vi "系统设置_古田污水厂.vi"() -> ()   [LabVIEW 2016]
uses:
  <vilib>/Utility/miscctls.llb/LVPointTypeDef.ctl
  <vilib>/Utility/config.llb/Read Key (U32).vi
  <vilib>/Utility/config.llb/Write Key (I32).vi
  PLC/PLC.lvlib
  <vilib>/ptbypt/NI_PtbyPt.lvlib
  <vilib>/Utility/config.llb/NI_LVConfig.lvlib
panel:
  out "循环次数":i32
  out "CODCr启动失败":bool
  out "输出簇":T1
  in  "运行模式":enum16{"维护模式", "常规模式", "应急模式", "质控模式"}(ring)
  in  "运行周期":i16=4 caption="运行间隔" min=1 max=24
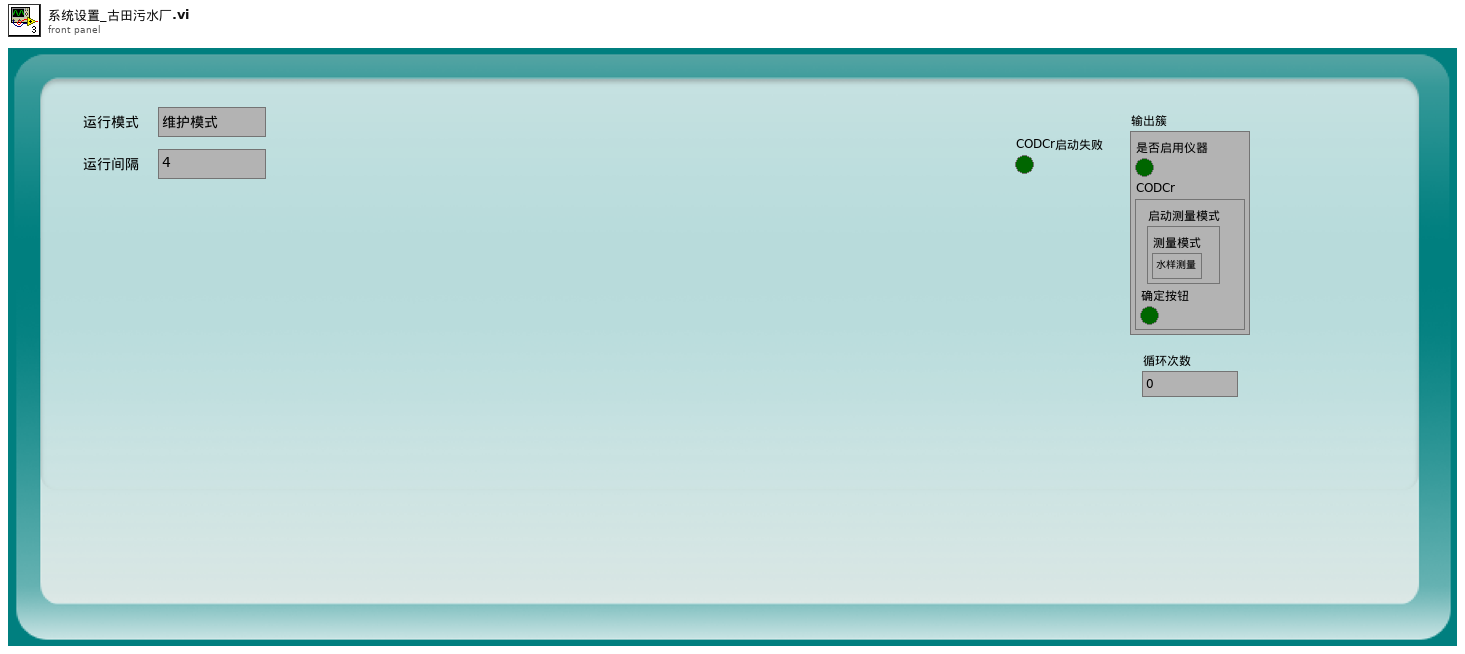
[diagram p1: front panel]
types:
  T1 = cluster{"是否启用仪器":bool, "CODCr":cluster{"启动测量模式":cluster{"测量模式":enum16{"水样测量", "标样核查", "零点核查", "加标回收", "平行样", "校零", "校标"}}, "确定按钮":bool}}
  T2 = typedef "LVPointTypeDef.ctl" = cluster{"Horizontal":i16, "Vertical":i16}
  T3 = typedef "NI_LVConfig.lvlib/Config Data RefNum.ctl" = refnum<k1>
  T4 = enum16{"水样测量", "标样核查", "零点核查", "加标回收", "平行样", "校零", "校标"}
  T5 = typedef "LVDateTimeRec.ctl" = cluster{"秒数的小数部分":dbl, "秒":i32, "分":i32, "时":i32, "日":i32, "月":i32, "年":i32, "天数（周）":i32, "天数（年）":i32, "DST":i32}
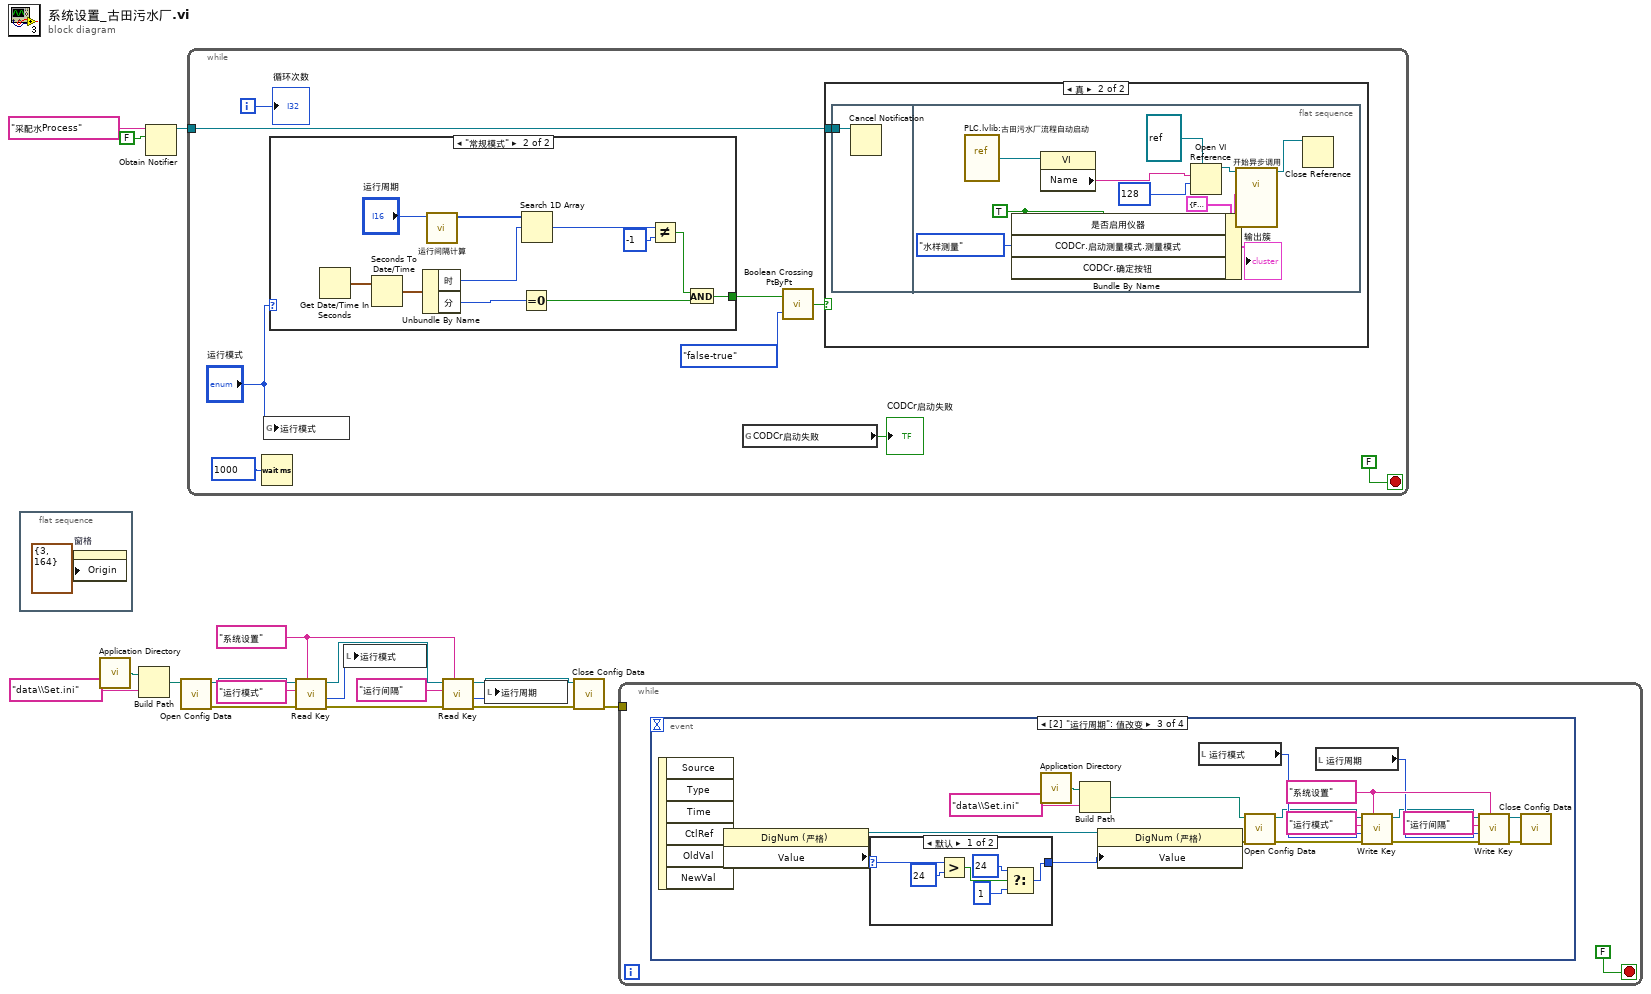
[diagram p0: block diagram]
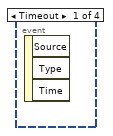
[diagram p4: hidden frame]
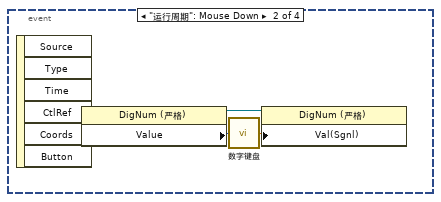
[diagram p5: hidden frame]
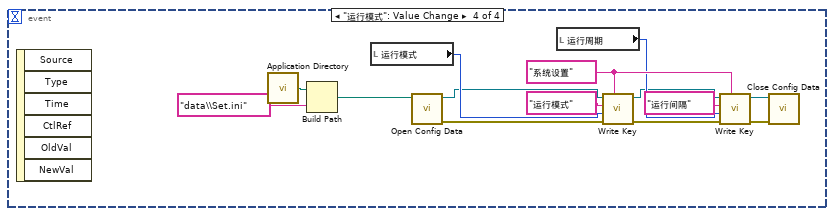
[diagram p7: hidden frame]
diagram:
  w2 = "系统设置" ("section")
  n1 = flat-sequence {
    frame #0 {
      n2 = property on="窗格" class="Pane"("Origin"=T2 {"Horizontal"=3, "Vertical"=164} ("原点")) -> ()  [unwired: 2 in, 2 out]
    }
  }
  n3 = call <vilib>:"Application Directory.vi"() -> ("Application Directory"=w13:path)
  n4 = Build Path(base path=w13, name or relative path="data\\Set.ini" ("名称或相对路径")) -> (appended path=w11:path)
  n5 = Obtain Notifier(name (unnamed)="采配水Process" ("名称（未命名）"), notification data type=FALSE) -> (notifier out=w16:refnum<notifier>)  [unwired: 2 in, 2 out]
  n6 = call <vilib>:"Open Config Data.vi"("configuration file path"=w11) -> ("error out"=w14:errorcluster, "refnum"=w15:T3)  [unwired: 8 in, 1 out]
  n7 = while {
    tunnel: w16 -> [w26]
    i -> [w20]
    stop <- FALSE stop-if-true
    n8 = Wait (ms)(milliseconds to wait=u32 1000 ("等待时间（毫秒）")) -> ()  [unwired: 1 out]
    n9 = global write "系统变量.vi" "运行模式"("运行模式") -> ()
    n10 = case shown="\"常规模式\"" "运行模式" {
      tunnel: [_ w41] -> w25
      frame "维护模式", Default {
      }
      frame "常规模式" {
        n11 = Get Date/Time In Seconds() -> (seconds since 1Jan1904=w50:timestamp)
        n12 = Seconds To Date/Time(time stamp (now)=w50) -> (date time rec=w49:T5)  [unwired: 1 in]
        n13 = Unbundle By Name(w49) -> ("时"=w46:i32, "分"=w48:i32)
        n14 = call "运行间隔计算.vi"("运行周期"="运行周期") -> ("数组"=w47:i32[])  [unwired: 10 in]
        n15 = Equal To 0?(x=w48) -> (x = 0?=w42:bool)
        n16 = Search 1D Array(1D array=w47, element=w46) -> (index of element=w45:i32)  [unwired: 1 in]
        n17 = Not Equal?(x=w45, y=-1) -> (x != y?=w43:bool)
        n18 = And(x=w43, y=w42) -> (x .and. y?=w41:bool)
      }
    }
    n19 = global read "系统变量.vi" "CODCr启动失败"() -> (→"CODCr启动失败":bool)
    n20 = call <vilib>:"Boolean Crossing PtByPt.vi"("direction"=enum16{"either", "false-true", "true-false"}."false-true", "input"=w25) -> ("crossing"=w23:bool)  [unwired: 1 in]
    n21 = case shown="真" w23 {
      tunnel: w26 -> [_ w29]
      frame False {
      }
      frame True {
        n22 = flat-sequence {
          tunnel: w29 -> [w30]
          frame #0 {
            n23 = Cancel Notification(0:w30) -> ()  [unwired: 1 in, 3 out]
          }
          frame #1 {
            w38 = TRUE ("是否启用仪器")
            n24 = vi-ref "PLC.lvlib:古田污水厂流程自动启动.vi"() -> (w32:refnum<vi>)
            n25 = Bundle By Name(cluster=T1 {"是否启用仪器"=FALSE, "CODCr"={"启动测量模式"={"测量模式"=enum."水样测量"}, "确定按钮"=TRUE}} ("参数"), "是否启用仪器"=w38, "CODCr.启动测量模式.测量模式"=T4."水样测量", "CODCr.确定按钮"=w38) -> (w33:T1)
            "输出簇" <- w33
            n26 = property class="VI"(reference=w32) -> ("Name"=w31:string)  [unwired: 1 in, 2 out]
            n27 = Open VI Reference(type specifier VI Refnum (for type only)=refnum<vi> refnum ("类型说明符VI引用句柄（仅用于类型）"), vi path=w31, options=128 ("选项")) -> (vi reference=w36:refnum<vi>)  [unwired: 3 in, 1 out]
            n28 = call-by-ref "开始异步调用"(reference=w36, "参数"=w33) -> (reference out=w35:refnum<vi>)  [unwired: 11 in, 2 out]
            n29 = Close Reference(reference=w35) -> ()  [unwired: 1 in, 1 out]
          }
        }
      }
    }
    "循环次数" <- w20
  }
  n30 = call-poly <vilib>:"Read Key.vi"("section"=w2, "error in (no error)"=w14, "key"="运行模式" ("section"), "refnum"=w15) -> ("error out"=w7:errorcluster, "value"=w10:u32, "refnum out"=w9:T3)  [unwired: 4 in, 1 out]
  n31 = local write "运行模式"(w10) -> ()
  n32 = call-poly <vilib>:"Read Key.vi"("section"=w2, "error in (no error)"=w7, "key"="运行间隔" ("section"), "refnum"=w9) -> ("error out"=w6:errorcluster, "value"=w3:u32, "refnum out"=w8:T3)  [unwired: 4 in, 1 out]
  n33 = local write "运行周期"(w3) -> ()
  n34 = call <vilib>:"Close Config Data.vi"("error in (no error)"=w6, "refnum"=w8) -> ("error out"=w1:errorcluster)  [unwired: 8 in, 1 out]
  n35 = while {
    tunnel: w1 -> [_]
    stop <- FALSE stop-if-true
    n36 = event shown="[2] \"运行周期\": 值改变" {
      selector: _ -> [_ _ _ _]
      dyn-events: _ -> [_ _ _ _]
      timeout: _ -> [_ _ _ _]
      event Timeout {
        n37 = event-data() -> ()  [unwired: 1 in, 3 out]
      }
      event "运行周期": Mouse Down {
        n38 = event-data() -> ("CtlRef"=w53:refnum<vi>)  [unwired: 1 in, 5 out]
        n39 = property class="DigNum (严格)"(reference=w53) -> (reference out=w55:refnum<vi>, "Value"=w54:i16)  [unwired: 1 in, 1 out]
        n40 = call "数字键盘.vi"("OldNumber"=w54) -> ("NewNumber"=w56:sgl)
        n41 = property class="DigNum (严格)"(reference=w55, "Val(Sgnl)"=w56) -> ()  [unwired: 1 in, 2 out]
      }
      event "运行周期": Value Change {
        w71 = "系统设置" ("section")
        n42 = event-data() -> ("CtlRef"=w75:refnum<vi>)  [unwired: 1 in, 5 out]
        n43 = property class="DigNum (严格)"(reference=w75) -> (reference out=w73:refnum<vi>, "Value"=w74:i16)  [unwired: 1 in, 1 out]
        n44 = case shown="默认" w74 {
          selector: w74 -> [w78 w82]
          tunnel: [w77 w82] -> w72
          frame Default {
            n45 = Greater?(x=w78, y=i16 24) -> (0:w80:bool)
            n46 = Select(t=i16 24 ("y"), s=w80, f=i16 1) -> (s? t:f=w77:i16)
          }
          frame 1..24 {
          }
        }
        n47 = call <vilib>:"Application Directory.vi"() -> ("Application Directory"=w66:path)
        n48 = Build Path(base path=w66, name or relative path="data\\Set.ini" ("名称或相对路径")) -> (appended path=w64:path)
        n49 = property class="DigNum (严格)"(reference=w73, "Value"=w72) -> (error out=w57:errorcluster)  [unwired: 1 in, 1 out]
        n50 = local read "运行模式"() -> (w69:enum16{"维护模式", "常规模式", "应急模式", "质控模式"})
        n51 = call <vilib>:"Open Config Data.vi"("error in (no error)"=w57, "configuration file path"=w64) -> ("error out"=w67:errorcluster, "refnum"=w68:T3)  [unwired: 7 in, 1 out]
        n52 = local read "运行周期"() -> (w70:i16)
        n53 = call-poly <vilib>:"Write Key.vi"("section"=w71, "error in (no error)"=w67, "value"=w69, "key"="运行模式" ("section"), "refnum"=w68) -> ("error out"=w61:errorcluster, "refnum out"=w63:T3)  [unwired: 4 in, 1 out]
        n54 = call-poly <vilib>:"Write Key.vi"("section"=w71, "error in (no error)"=w61, "value"=w70, "key"="运行间隔" ("section"), "refnum"=w63) -> ("error out"=w60:errorcluster, "refnum out"=w62:T3)  [unwired: 4 in, 1 out]
        n55 = call <vilib>:"Close Config Data.vi"("error in (no error)"=w60, "refnum"=w62) -> ()  [unwired: 8 in, 2 out]
      }
      event "运行模式": Value Change {
        w96 = "系统设置" ("section")
        n56 = event-data() -> ()  [unwired: 1 in, 6 out]
        n57 = call <vilib>:"Application Directory.vi"() -> ("Application Directory"=w91:path)
        n58 = Build Path(base path=w91, name or relative path="data\\Set.ini" ("名称或相对路径")) -> (appended path=w89:path)
        n59 = local read "运行模式"() -> (w94:enum16{"维护模式", "常规模式", "应急模式", "质控模式"})
        n60 = call <vilib>:"Open Config Data.vi"("configuration file path"=w89) -> ("error out"=w92:errorcluster, "refnum"=w93:T3)  [unwired: 8 in, 1 out]
        n61 = local read "运行周期"() -> (w95:i16)
        n62 = call-poly <vilib>:"Write Key.vi"("section"=w96, "error in (no error)"=w92, "value"=w94, "key"="运行模式" ("section"), "refnum"=w93) -> ("error out"=w86:errorcluster, "refnum out"=w88:T3)  [unwired: 4 in, 1 out]
        n63 = call-poly <vilib>:"Write Key.vi"("section"=w96, "error in (no error)"=w86, "value"=w95, "key"="运行间隔" ("section"), "refnum"=w88) -> ("error out"=w85:errorcluster, "refnum out"=w87:T3)  [unwired: 4 in, 1 out]
        n64 = call <vilib>:"Close Config Data.vi"("error in (no error)"=w85, "refnum"=w87) -> ()  [unwired: 8 in, 2 out]
      }
    }
  }
